vi "Behaviour Tree.vi"(11 "IO":T1) -> (3 "bt_Node out":refnum<class "bt_Node.lvclass">)   [LabVIEW 2021, in "Test Sequencer Support.lvlib"]
uses:
  Test Sequencer Support.lvlib
  Support/Nodes/abs_Node/bt_Node.lvclass
  IO Type.ctl
  <vilib>/TSA/Event Log/Event_TextLog/Event_TextLog.lvclass
  Blackboard/Blackboard.lvclass
  <vilib>/TSA/Abstract Data Classes/Abs_Types/Boolean/Abs_Boolean.lvclass
  <vilib>/TSA/Abstract Data Classes/Abs_Types/Waveform/Abs_Waveform.lvclass
  <vilib>/TSA/Abstract Data Classes/Abs_Types/Double Float/Abs_Double Float.lvclass
  Support/Nodes/Decorators/Repeater/Support/Finish On - Type.ctl
  BT.lvlib
  Support/Nodes/Decorators/Repeater/bt_Repeater.lvclass
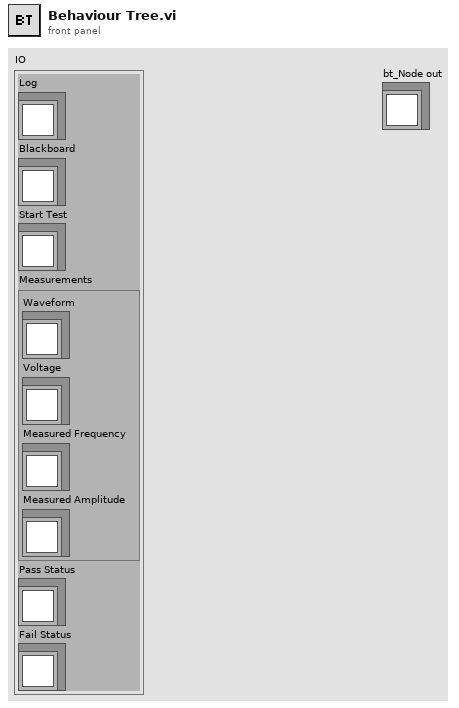
[diagram p1: front panel]
types:
  T1 = typedef "Test Sequencer Support.lvlib/IO Type.ctl" = cluster{"Log":refnum<class "Event_TextLog.lvclass">, "Blackboard":refnum<class "Blackboard.lvclass">, "Start Test":refnum<class "Abs_Boolean.lvclass">, "Measurements":cluster{"Waveform":refnum<class "Abs_Waveform.lvclass">, "Voltage":refnum<class "Abs_Double Float.lvclass">, "Measured Frequency":refnum<class "Abs_Double Float.lvclass">, "Measured Amplitude":refnum<class "Abs_Double Float.lvclass">}, "Pass Status":refnum<class "Abs_Boolean.lvclass">, "Fail Status":refnum<class "Abs_Boolean.lvclass">}
  T2 = typedef "BT.lvlib/bt_Repeater.lvclass/Finish On - Type.ctl" = enum16{"Success", "Failure", "Never"}
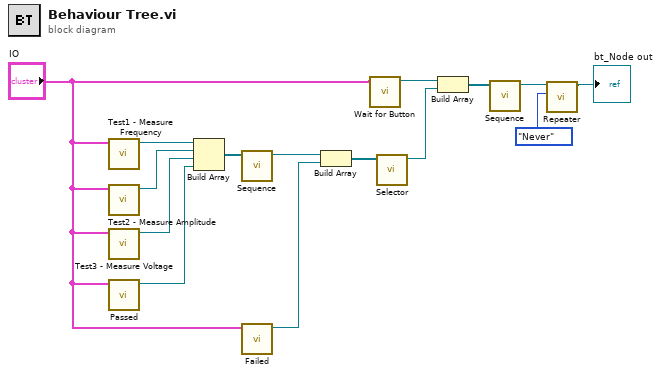
[diagram p0: block diagram]
diagram:
  n1 = call "Test1 - Measure Frequency.vi"("IO"="IO") -> ("Node"=w7:refnum<class "bt_Node.lvclass">)  [unwired: 10 in]
  n2 = call "Test2 - Measure Amplitude.vi"("IO"="IO") -> ("Node"=w4:refnum<class "bt_Node.lvclass">)  [unwired: 10 in]
  n3 = call "Test3 - Measure Voltage.vi"("IO"="IO") -> ("Node"=w5:refnum<class "bt_Node.lvclass">)  [unwired: 10 in]
  n4 = call "Passed.vi"("IO"="IO") -> ("Node"=w3:refnum<class "bt_Node.lvclass">)  [unwired: 10 in]
  n5 = Build Array(w7, w4, w5, w3) -> (w8:refnum<class "bt_Node.lvclass">[])
  n6 = call "Sequence.vi"("Nodes"=w8) -> ("Node"=w10:refnum<class "bt_Node.lvclass">)  [unwired: 10 in]
  n7 = call "Failed.vi"("IO"="IO") -> ("Node"=w2:refnum<class "bt_Node.lvclass">)  [unwired: 10 in]
  n8 = Build Array(w10, w2) -> (w9:refnum<class "bt_Node.lvclass">[])
  n9 = call "Wait for Button.vi"("IO"="IO") -> ("bt_Node out"=w6:refnum<class "bt_Node.lvclass">)  [unwired: 10 in]
  n10 = call "Selector.vi"("Nodes"=w9) -> ("Node"=w11:refnum<class "bt_Node.lvclass">)  [unwired: 10 in]
  n11 = Build Array(w6, w11) -> (w12:refnum<class "bt_Node.lvclass">[])
  n12 = call "Sequence.vi"("Nodes"=w12) -> ("Node"=w13:refnum<class "bt_Node.lvclass">)  [unwired: 10 in]
  n13 = call "Repeater.vi"("Finish On"=Finish_On_-_Type."Never", "Node In"=w13) -> ("Node Out"=→"bt_Node out":refnum<class "bt_Node.lvclass">)  [unwired: 9 in]
